vi "Main.vi"() -> ()   [LabVIEW 2020]
doc: "This template is for the Queued Message Handler design pattern.\n\nThe Event Handling Loop generates messages based on user interface actions.\n\nThe Message Handling Loop processes messages generated by the Event Handling Loop, or by other messages. The messages are string values, so new messages can be added easily to the Message Cases case structure in the Message Handling Loop. Each message cluster can also provide an optional value for Message Data, which is a variant that can be converted to whatever message-specific data is required."
uses:
  controls/UI Data.ctl
  classes/Scheduled Enqueue/Scheduled Enqueue.lvclass
  support/Message Queue/Enqueue Message (Single).vi
  <vilib>/Utility/error.llb/Error Cluster From Error Code.vi
  <vilib>/ErrorRing/Error Ring.xnode
  support/Message Queue/Message Queue.lvlib
  support/User Event - Stop/User Event - Stop.lvlib
panel:
  out "current time":timestamp format="%<%.3X>T"
  out "Auto-Save":bool
  in  "Auto-Save Period (s)":dbl=5.0 min=1.0
  in  "Toggle Auto Save":bool
  out "Display":string
  in  "Do Something Else <Replace Me>":bool
  in  "Do Something <Replace Me>":bool
  in  "Exit":bool
  # "These controls have associated \"Value Changed\" events configured in the Event Structure on the diagram.\n\nReplace them (and reconfigure the Event Structure) with the controls you need for your application."
  # "This template is for the Queued Message Handler design pattern.\n\nSee the block diagram for more information on how to use this template."
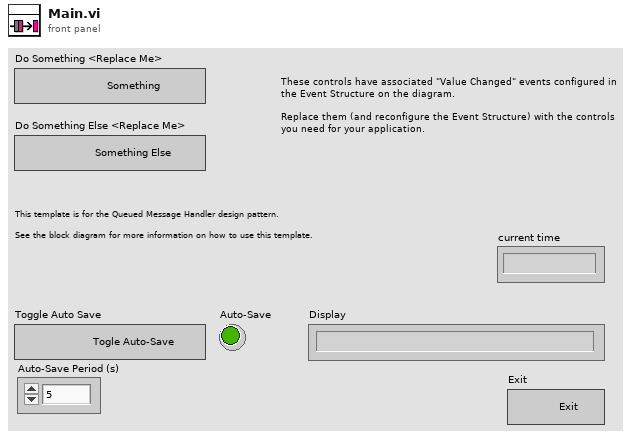
[diagram p1: front panel]
types:
  T1 = typedef "UI Data.ctl" = cluster{"AutoSave":bool, "SchedEnqueue":refnum<class "Scheduled Enqueue.lvclass">}
  T2 = typedef "Message Queue.lvlib/All Message Queues.ctl" = cluster{"UI":refnum<queue>}
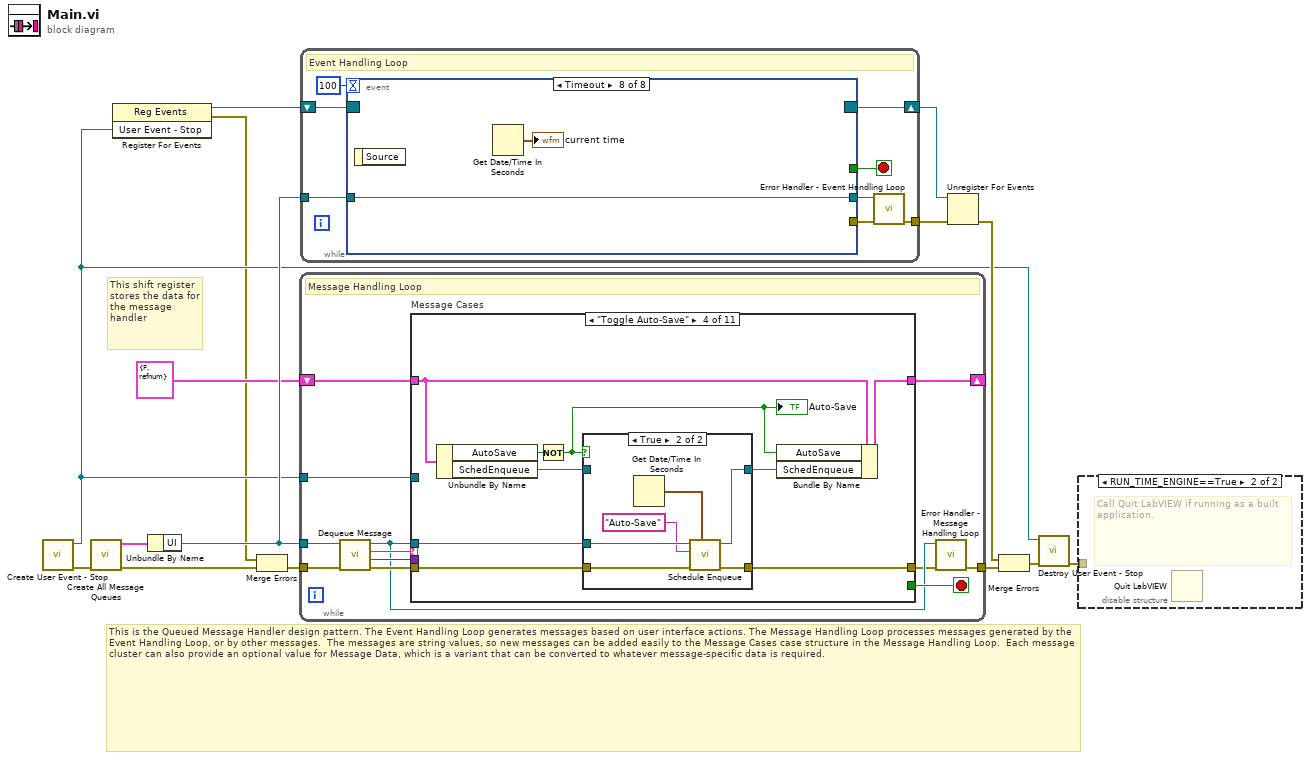
[diagram p0: block diagram]
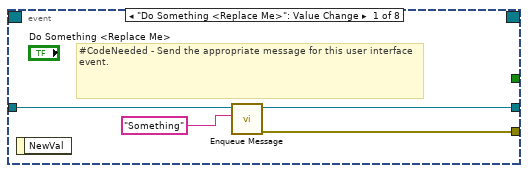
[diagram p3: hidden frame]
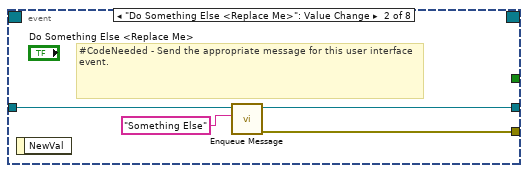
[diagram p4: hidden frame]
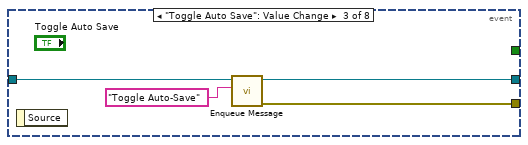
[diagram p5: hidden frame]
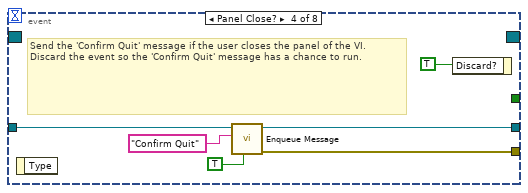
[diagram p6: hidden frame]
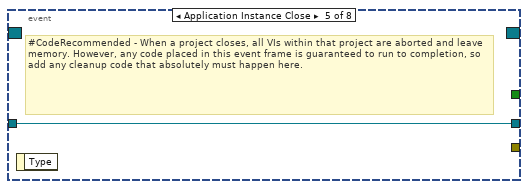
[diagram p7: hidden frame]
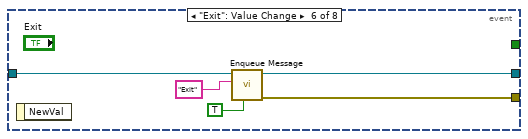
[diagram p8: hidden frame]
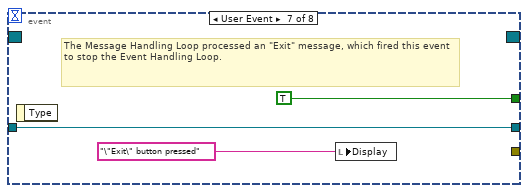
[diagram p9: hidden frame]
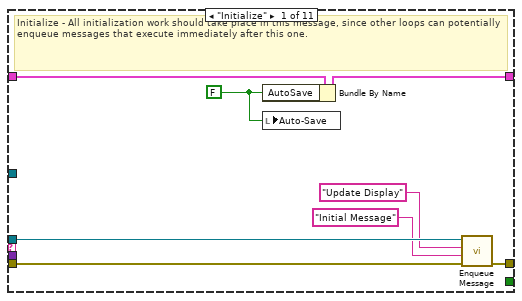
[diagram p10: hidden frame]
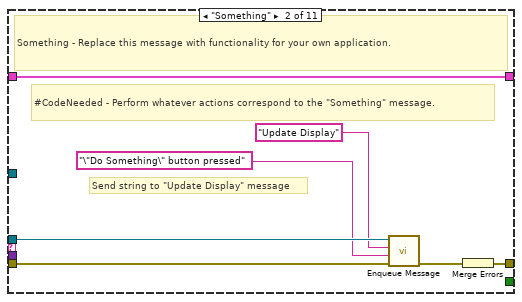
[diagram p11: hidden frame]
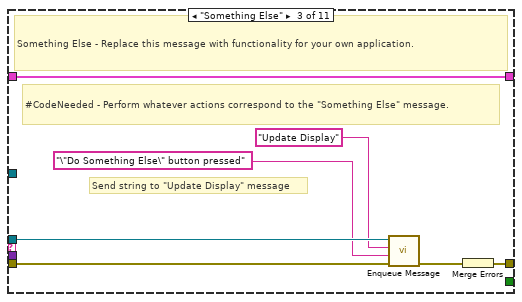
[diagram p12: hidden frame]
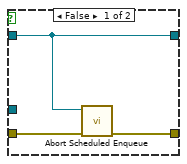
[diagram p13: hidden frame]
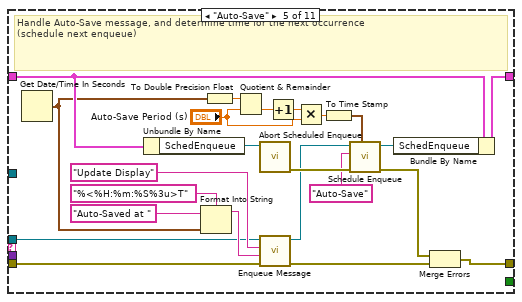
[diagram p14: hidden frame]
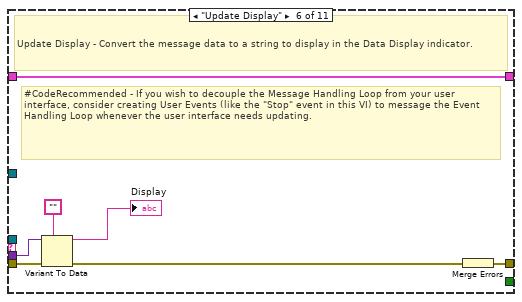
[diagram p15: hidden frame]
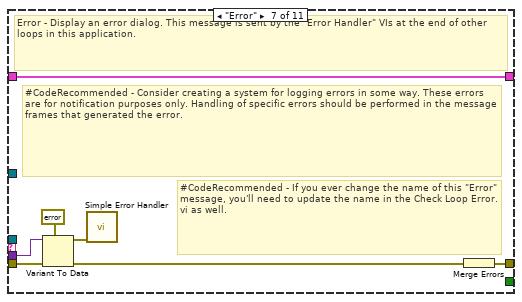
[diagram p16: hidden frame]
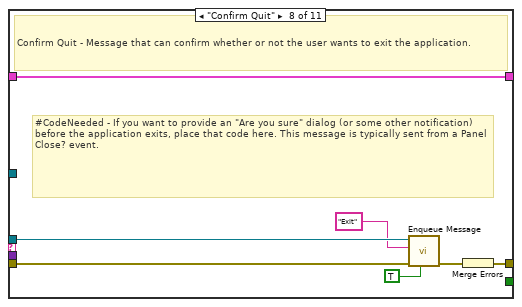
[diagram p17: hidden frame]
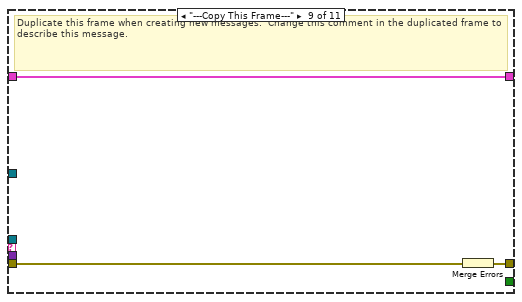
[diagram p18: hidden frame]
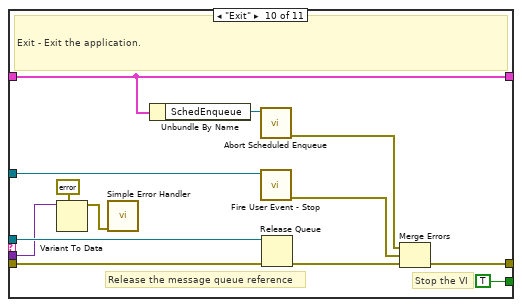
[diagram p19: hidden frame]
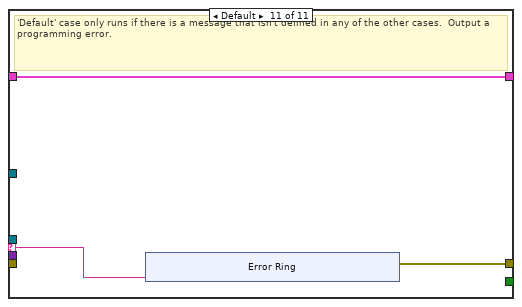
[diagram p20: hidden frame]
diagram:
  # "This is the Queued Message Handler design pattern. The Event Handling Loop generates messages based on user interface actions. The Message Handling Loop processes messages generated by the Event Handling Loop, or by other messages.  The messages are string values, so new messages can be added easily to the Message Cases case structure in the Message Handling Loop.  Each message cluster can also provide an optional value for Message Data, which is a variant that can be converted to whatever message-specific data is required."
  # "This shift register stores the data for the message handler"
  n1 = call "Create User Event - Stop.vi"() -> ("error out"=w11:errorcluster, "User Event - Stop"=w3:refnum<user-event>)  [unwired: 10 in]
  n2 = call "Create All Message Queues.vi"("error in (no error)"=w11) -> ("error out"=w15:errorcluster, "Message Queues out"=w14:T2)  [unwired: 9 in]
  n3 = register-events(w3) -> (reference out=w4:refnum<event-registration>, error out=w1:errorcluster)  [unwired: 2 in]
  n4 = Unbundle By Name(w14) -> ("UI"=w12:refnum<queue>)
  n5 = Merge Errors(w1, w15) -> (w2:errorcluster)
  n6 = while {
    tunnel: w12 -> [w19]
    shift-right: [w26] -> _
    shift-left: T1 {"AutoSave"=FALSE, "SchedEnqueue"=refnum} ("Data Cluster") -> [w27]
    tunnel: w3 -> [w24]
    tunnel: w2 -> [w23]
    tunnel: [w17] -> w13
    stop <- w25 stop-if-true
    # "Message Handling Loop"
    n7 = call "Dequeue Message.vi"("error in (no error)"=w23, "Message Queue"=w19) -> ("error out"=w22:errorcluster, "Message Data"=w20:variant, "Message"=w21:string, "dup Message Queue"=w18:refnum<queue>)  [unwired: 6 in]
    n8 = case "Message Cases" shown="\"Toggle Auto-Save\"" w21 {
      selector: w21 -> [_ _ _ _ _ _ _ _ _ _ w128]
      tunnel: w18 -> [w35 w38 w45 w56 w74 _ _ w107 _ w127 _]
      tunnel: w22 -> [w33 w40 w47 w55 w73 w95 w104 w111 w114 w121 _]
      tunnel: [w34 w41 w48 w54 w72 w96 w98 w109 w112 w124 w129] -> w16
      tunnel: w27 -> [w32 w42 w49 w58 w86 w97 w103 w110 w113 w117 w130]
      tunnel: [w29 w42 w49 w53 w83 w97 w103 w110 w113 w117 w130] -> w26
      tunnel: [_ _ _ _ _ _ _ _ _ TRUE _] -> w25
      tunnel: w20 -> [_ _ _ _ _ w94 w102 _ _ w118 _]
      tunnel: w24 -> [_ _ _ _ _ _ _ _ _ w123 _]
      frame "Initialize" {
        w28 = FALSE ("AutoSave")
        # "Initialize - All initialization work should take place in this message, since other loops can potentially enqueue messages that execute immediately after this one."
        n9 = Bundle By Name(cluster=w32, "AutoSave"=w28) -> (w29:T1)
        n10 = local write "Auto-Save"(w28) -> ()
        n11 = call-poly "Enqueue Message.vi"("error in (no error)"=w33, "Message Data"="Initial Message" ("Initial Message"), "Message"="Update Display", "Message Queue"=w35) -> ("error out"=w34:errorcluster)  [unwired: 6 in, 1 out]
      }
      frame "Something" {
        # "Send string to \"Update Display\" message"
        # "#CodeNeeded - Perform whatever actions correspond to the \"Something\" message."
        # "Something - Replace this message with functionality for your own application."
        n12 = call-poly "Enqueue Message.vi"("error in (no error)"=w40, "Message Data"="\"Do Something\" button pressed" ("\"Do Something\" button pressed"), "Message"="Update Display", "Message Queue"=w38) -> ("error out"=w39:errorcluster)  [unwired: 6 in, 1 out]
        n13 = Merge Errors(w39) -> (w41:errorcluster)
      }
      frame "Something Else" {
        # "Send string to \"Update Display\" message"
        # "#CodeNeeded - Perform whatever actions correspond to the \"Something Else\" message."
        # "Something Else - Replace this message with functionality for your own application."
        n14 = call-poly "Enqueue Message.vi"("error in (no error)"=w47, "Message Data"="\"Do Something Else\" button pressed" ("\"Do Something Else\" button pressed"), "Message"="Update Display", "Message Queue"=w45) -> ("error out"=w46:errorcluster)  [unwired: 6 in, 1 out]
        n15 = Merge Errors(w46) -> (w48:errorcluster)
      }
      frame "Toggle Auto-Save" {
        n16 = Unbundle By Name(w58) -> ("AutoSave"=w51:bool, "SchedEnqueue"=w57:refnum<class "Scheduled Enqueue.lvclass">)
        n17 = Not(x=w51) -> (.not. x?=w50:bool)
        "Auto-Save" <- w50
        n18 = case shown="True" w50 {
          tunnel: w57 -> [w59 _]
          tunnel: w56 -> [_ w66]
          tunnel: w55 -> [w61 w65]
          tunnel: [w60 w64] -> w54
          tunnel: [w59 w62] -> w52
          frame False {
            n19 = call "Abort Scheduled Enqueue.vi"("error in (no error)"=w61, "Scheduled Message in"=w59) -> ("error out"=w60:errorcluster)  [unwired: 9 in]
          }
          frame True {
            n20 = Get Date/Time In Seconds() -> (seconds since 1Jan1904=w67:timestamp)
            n21 = call "Schedule Enqueue.vi"("StartTime"=w67, "error in (no error)"=w65, "Message"="Auto-Save", "Queue"=w66) -> ("error out"=w64:errorcluster, "Scheduled Enqueuer out"=w62:refnum<class "Scheduled Enqueue.lvclass">)  [unwired: 6 in]
          }
        }
        n22 = Bundle By Name(cluster=w58, "AutoSave"=w50, "SchedEnqueue"=w52) -> (w53:T1)
      }
      frame "Auto-Save" {
        # "Handle Auto-Save message, and determine time for the next occurrence\n(schedule next enqueue)"
        n23 = Get Date/Time In Seconds() -> (seconds since 1Jan1904=w70:timestamp)
        n24 = Unbundle By Name(w86) -> ("SchedEnqueue"=w85:refnum<class "Scheduled Enqueue.lvclass">)
        n25 = Format Into String(format string="%<%H:%m:%S%3u>T" ("\"Do Something\" button pressed"), initial string="Auto-Saved at ", w70) -> (resulting string=w88:string)  [unwired: 1 in, 1 out]
        n26 = To Double Precision Float(number=w70) -> (double precision float=w81:dbl)
        n27 = Quotient & Remainder(x=w81, y="Auto-Save Period (s)") -> (floor(x/y)=w79:dbl)  [unwired: 1 out]
        n28 = call "Abort Scheduled Enqueue.vi"("Scheduled Message in"=w85) -> ("error out"=w84:errorcluster)  [unwired: 10 in]
        n29 = call-poly "Enqueue Message.vi"("error in (no error)"=w73, "Message Data"=w88, "Message"="Update Display", "Message Queue"=w74) -> ("error out"=w90:errorcluster, "dup Message Queue"=w75:refnum<queue>)  [unwired: 6 in]
        n30 = Increment(x=w79) -> (x+1=w78:dbl)
        n31 = Multiply(x=w78, y="Auto-Save Period (s)") -> (x*y=w77:dbl)
        n32 = To Time Stamp(1:w77) -> (0:w76:timestamp)
        n33 = call "Schedule Enqueue.vi"("StartTime"=w76, "error in (no error)"=w84, "Message"="Auto-Save", "Queue"=w75) -> ("error out"=w71:errorcluster, "Scheduled Enqueuer out"=w82:refnum<class "Scheduled Enqueue.lvclass">)  [unwired: 6 in]
        n34 = Bundle By Name(cluster=w86, "SchedEnqueue"=w82) -> (w83:T1)
        n35 = Merge Errors(w71, w90) -> (w72:errorcluster)
      }
      frame "Update Display" {
        # "#CodeRecommended - If you wish to decouple the Message Handling Loop from your user interface, consider creating User Events (like the \"Stop\" event in this VI) to message the Event Handling Loop whenever the user interface needs updating."
        # "Update Display - Convert the message data to a string to display in the Data Display indicator."
        n36 = Variant To Data(error in=w95, type="", Variant=w94) -> (data=→"Display":string, error out=w92:errorcluster)
        n37 = Merge Errors(w92) -> (w96:errorcluster)
      }
      frame "Error" {
        # "#CodeRecommended - If you ever change the name of this \"Error\" message, you'll need to update the name in the Check Loop Error.vi as well."
        # "#CodeRecommended - Consider creating a system for logging errors in some way. These errors are for notification purposes only. Handling of specific errors should be performed in the message frames that generated the error."
        # "Error - Display an error dialog. This message is sent by the \"Error Handler\" VIs at the end of other loops in this application."
        n38 = Variant To Data(error in=w104, type=errorcluster {"status"=FALSE, "code"=0, "source"=""} ("error constant"), Variant=w102) -> (data=w100:errorcluster, error out=w99:errorcluster)
        n39 = call <vilib>:"Simple Error Handler.vi"("error in (no error)"=w100) -> ()  [unwired: 4 in, 5 out]
        n40 = Merge Errors(w99) -> (w98:errorcluster)
      }
      frame "Confirm Quit" {
        # "#CodeNeeded - If you want to provide an \"Are you sure\" dialog (or some other notification) before the application exits, place that code here. This message is typically sent from a Panel Close? event."
        # "Confirm Quit - Message that can confirm whether or not the user wants to exit the application."
        n41 = call-poly "Enqueue Message.vi"("Priority Message? (F)"=TRUE, "error in (no error)"=w111, "Message"="Exit", "Message Queue"=w107) -> ("error out"=w108:errorcluster)  [unwired: 6 in, 1 out]
        n42 = Merge Errors(w108) -> (w109:errorcluster)
      }
      frame "---Copy This Frame---" {
        # "Duplicate this frame when creating new messages.  Change this comment in the duplicated frame to describe this message."
        n43 = Merge Errors(w114) -> (w112:errorcluster)
      }
      frame "Exit" {
        # "Stop the VI"
        # "Release the message queue reference"
        # "Exit - Exit the application."
        n44 = Variant To Data(type=errorcluster {"status"=FALSE, "code"=0, "source"=""} ("error constant"), Variant=w118) -> (data=w119:errorcluster)  [unwired: 1 in, 1 out]
        n45 = call <vilib>:"Simple Error Handler.vi"("error in (no error)"=w119) -> ()  [unwired: 4 in, 5 out]
        n46 = Unbundle By Name(w117) -> ("SchedEnqueue"=w116:refnum<class "Scheduled Enqueue.lvclass">)
        n47 = call "Abort Scheduled Enqueue.vi"("Scheduled Message in"=w116) -> ("error out"=w115:errorcluster)  [unwired: 10 in]
        n48 = call "Fire User Event - Stop.vi"("User Event - Stop"=w123) -> ("error out"=w122:errorcluster)  [unwired: 10 in]
        n49 = Release Queue(queue=w127, error in (no error)=w121) -> (error out=w125:errorcluster)  [unwired: 1 in, 2 out]
        n50 = Merge Errors(w115, w122, w125) -> (w124:errorcluster)
      }
      frame Default {
        # "'Default' case only runs if there is a message that isn't defined in any of the other cases.  Output a programming error."
        n51 = xnode "Error Ring"("parameter 0"=w128) -> ("error out"=w129:errorcluster)
      }
    }
    n52 = call "Error Handler - Message Handling Loop.vi"("error in (no error)"=w16, "Message Queue"=w18) -> ("dup error in"=w17:errorcluster)  [unwired: 8 in, 1 out]
  }
  n53 = while {
    tunnel: w12 -> [w145]
    shift-right: [w143] -> w8
    shift-left: w4 -> [w144]
    tunnel: [w139] -> w5
    stop <- w141 stop-if-true
    # "Event Handling Loop"
    n54 = event shown="[7] Timeout" {
      selector: w144 -> [_ _ _ _ _ _ _ _]
      dyn-events: [_ _ _ _ _ _ _ _] -> w143
      timeout: 100 -> [_ _ _ _ _ _ _ _]
      tunnel: [_ _ _ _ _ _ TRUE ("Discard?") _] -> w141
      tunnel: w145 -> [w149 w153 w156 w162 w164 w169 w172 w174]
      tunnel: [w146 w150 w154 w161 _ w168 _ _] -> w142
      tunnel: [w148 w152 w155 w160 w164 w167 w172 w174] -> w140
      event "Do Something <Replace Me>": Value Change {
        # "#CodeNeeded - Send the appropriate message for this user interface event."
        n55 = event-data() -> ()  [unwired: 1 in, 1 out]
        n56 = call-poly "Enqueue Message.vi"("Message"="Something", "Message Queue"=w149) -> ("error out"=w146:errorcluster, "dup Message Queue"=w148:refnum<queue>)  [unwired: 8 in]
      }
      event "Do Something Else <Replace Me>": Value Change {
        # "#CodeNeeded - Send the appropriate message for this user interface event."
        n57 = event-data() -> ()  [unwired: 1 in, 1 out]
        n58 = call-poly "Enqueue Message.vi"("Message"="Something Else", "Message Queue"=w153) -> ("error out"=w150:errorcluster, "dup Message Queue"=w152:refnum<queue>)  [unwired: 8 in]
      }
      event "Toggle Auto Save": Value Change {
        n59 = event-data() -> ()  [unwired: 1 in, 1 out]
        n60 = call-poly "Enqueue Message.vi"("Message"="Toggle Auto-Save", "Message Queue"=w156) -> ("error out"=w154:errorcluster, "dup Message Queue"=w155:refnum<queue>)  [unwired: 8 in]
      }
      event Panel Close? {
        # "Send the 'Confirm Quit' message if the user closes the panel of the VI. Discard the event so the 'Confirm Quit' message has a chance to run."
        n61 = event-data() -> ()  [unwired: 1 in, 1 out]
        n62 = call-poly "Enqueue Message.vi"("Priority Message? (F)"=TRUE, "Message"="Confirm Quit", "Message Queue"=w162) -> ("error out"=w161:errorcluster, "dup Message Queue"=w160:refnum<queue>)  [unwired: 7 in]
        n63 = event-data("Discard?"=TRUE) -> ()  [unwired: 1 in, 1 out]
      }
      event Application Instance Close {
        # "#CodeRecommended - When a project closes, all VIs within that project are aborted and leave memory. However, any code placed in this event frame is guaranteed to run to completion, so add any cleanup code that absolutely must happen here."
        n64 = event-data() -> ()  [unwired: 1 in, 1 out]
      }
      event "Exit": Value Change {
        n65 = event-data() -> ()  [unwired: 1 in, 1 out]
        n66 = call-poly "Enqueue Message.vi"("Priority Message? (F)"=TRUE, "Message"="Exit", "Message Queue"=w169) -> ("error out"=w168:errorcluster, "dup Message Queue"=w167:refnum<queue>)  [unwired: 7 in]
      }
      event User Event {
        # "The Message Handling Loop processed an \"Exit\" message, which fired this event to stop the Event Handling Loop."
        n67 = event-data() -> ()  [unwired: 1 in, 1 out]
        n68 = local write "Display"("\"Exit\" button pressed" ("VI Stopped")) -> ()
      }
      event Timeout {
        n69 = event-data() -> ()  [unwired: 1 in, 1 out]
        n70 = Get Date/Time In Seconds() -> (seconds since 1Jan1904=→"current time":timestamp)
      }
    }
    n71 = call "Error Handler - Event Handling Loop.vi"("error in (no error)"=w142, "Message Queue"=w140) -> ("dup error in"=w139:errorcluster)  [unwired: 8 in, 1 out]
  }
  n72 = Unregister For Events(event registration refnum=w8, error in=w5) -> (error out=w9:errorcluster)
  n73 = Merge Errors(w9, w13) -> (w10:errorcluster)
  n74 = call "Destroy User Event - Stop.vi"("error in (no error)"=w10, "User Event - Stop"=w3) -> ("error out"=w6:errorcluster)  [unwired: 9 in]
  n75 = disable-structure shown="RUN_TIME_ENGINE==True" {
    disable-tunnel: w6 -> [_ _]
    frame condition #0 (active) {
    }
    frame condition #1 {
      # "Call Quit LabVIEW if running as a built application."
      n76 = Quit LabVIEW() -> ()  [unwired: 1 in]
    }
  }
